vi "图片显示实验.vi"   [LabVIEW 2011]
uses:
  <vilib>/STM32_DriverVI_Interface_F4/LCD/LCD_Init_F4.vi
types:
  T1 = enum8{"P0", "P1", "P2", "P3", "P4", "P5", "P6", "P7", "P8", "P9", "P10", "P11", "P12", "P13", "P14", "P15"}
  T2 = enum8{"Port_A", "Port_B", "Port_C", "Port_D", "Port_E", "Port_F", "Port_G"}
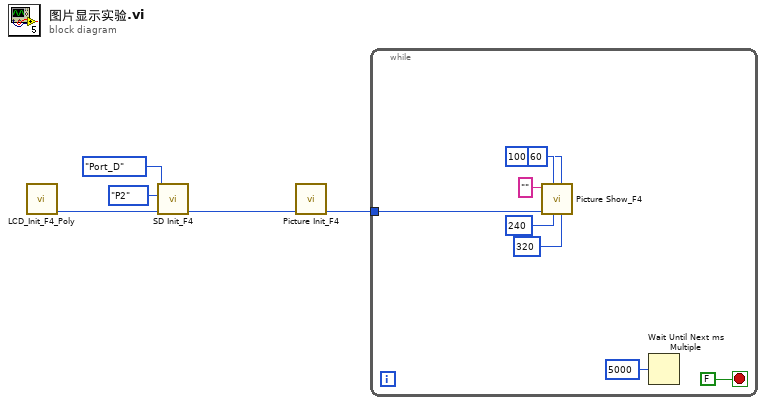
[diagram p0: block diagram]
diagram:
  n1 = call-poly <vilib>:"LCD_Init_F4_Poly.vi"() -> ("err_out"=w5:u8)  [unwired: 10 in, 1 out]
  n2 = call <vilib>:"SD Init_F4.vi"("err_in"=w5, "SD_CS_pin"=T1."P2", "SD_CS_PortX"=T2."Port_D") -> ("err_out"=w4:u8)  [unwired: 7 in, 1 out]
  n3 = call <vilib>:"Picture Init_F4.vi"("err_in"=w4) -> ("err_out"=w3:u8)  [unwired: 10 in]
  n4 = while {
    tunnel: w3 -> [w13]
    stop <- FALSE stop-if-true
    n5 = call <vilib>:"Picture Show_F4.vi"("Height"=u16 320, "Y_Position"=u16 60, "Width"=u16 240, "X_Position"=u16 100, "err_in"=w13, "Pic Path"="") -> ()  [unwired: 4 in, 2 out]
    n6 = Wait Until Next ms Multiple(millisecond multiple=u32 5000 ("毫秒倍数")) -> ()  [unwired: 1 out]
  }
